vi "String to 2D DBL.vi"(1 "String":string) -> (0 "DBL":dbl[][](array[numeric]))   [LabVIEW 2020, in "2601B.lvclass"]
uses:
  2601B.lvclass
  2601B.lvclass/2601B.ctl
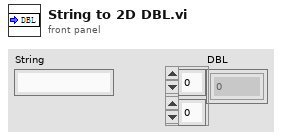
[diagram p1: front panel]
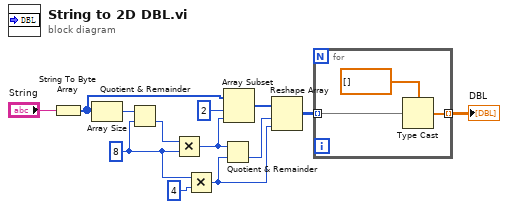
[diagram p0: block diagram]
diagram:
  w5 = 8 ("y")
  n1 = String To Byte Array(string="String") -> (unsigned byte array=w12:u8[])
  n2 = Array Size(array=w12) -> (size(s)=w6:i32)
  n3 = Quotient & Remainder(x=w6, y=w5) -> (floor(x/y)=w10:i32)  [unwired: 1 out]
  n4 = Multiply(x=w10, y=w5) -> (x*y=w3:i32)
  n5 = Multiply(x=w5, y=4 ("维数大小")) -> (x*y=w2:i32)
  n6 = Quotient & Remainder(x=w3, y=w2) -> (floor(x/y)=w1:i32)  [unwired: 1 out]
  n7 = Array Subset(array=w12, index=2 ("索引"), length=w3) -> (w8:u8[])
  n8 = Reshape Array(w8, w1, w2) -> (w11:u8[][])
  n9 = for {
    tunnel: [w16] -> w9 mode=indexing
    tunnel: w11 -> [w14] mode=indexing
    n10 = Type Cast(type=dbl[] [] ("*(类型 *) &x"), x=w14) -> (*(type *) &x=w16:dbl[])
  }
  "DBL" <- w9
